vi "SaveResultToMES.vi"(0 "class data in":refnum<class "CMESAPI.lvclass">, 5 "serialNumber":string, 7 "equipment":string, 11 "error in (no error)":errorcluster) -> (4 "class data out":refnum<class "CMESAPI.lvclass">, 6 "Result":bool, 15 "error out":errorcluster)   [LabVIEW 2020, in "Salcomp-MES.lvlib" / "CMESAPI.lvclass"]
uses:
  CMESAPI.lvclass
  <vilib>/gpm_packages/@cs/event-logger/Source/Composed Log/Types/Log Level.ctl
  CMESAPI.lvclass/CMESAPI.ctl
  E:/Git/Libraries/develop/CME-API/CMESAPI_Fw4.0_1.9.2/CMESAPI.dll
  CMESAPI_Fw4.0_1.9.2/CMESAPI.dll
  <vilib>/gpm_packages/@cs/event-logger/Source/Composed Log/LoggerReference/LoggerReference.lvclass/LoggerReference.ctl
  <vilib>/gpm_packages/@cs/event-logger/Source/Composed Log/LoggerReference/Log.vi
  <vilib>/gpm_packages/@cs/event-logger/Source/Composed Log/LoggerReference/Get Valid Event Time.vi
  <vilib>/gpm_packages/@cs/event-logger/Source/Composed Log/LoggerReference/Remove Stale Logs.vi
  <vilib>/gpm_packages/@cs/event-logger/Source/Composed Log/LoggerReference/LoggerReference.lvclass
  <vilib>/gpm_packages/@cs/event-logger/Source/Composed Log/Composed Log.lvlib
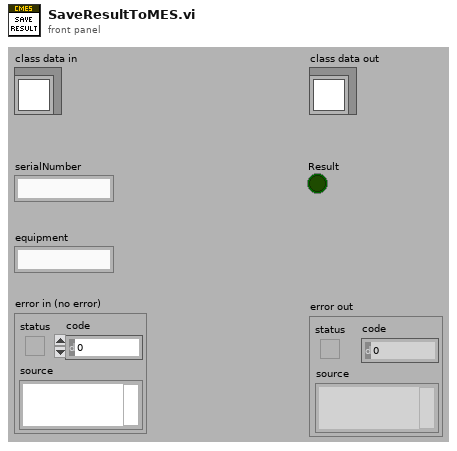
[diagram p1: front panel]
types:
  T1 = typedef "Composed Log.lvlib/Log Level.ctl" = enum16{"Debug", "Info", "Warning", "Error", "Critical"}
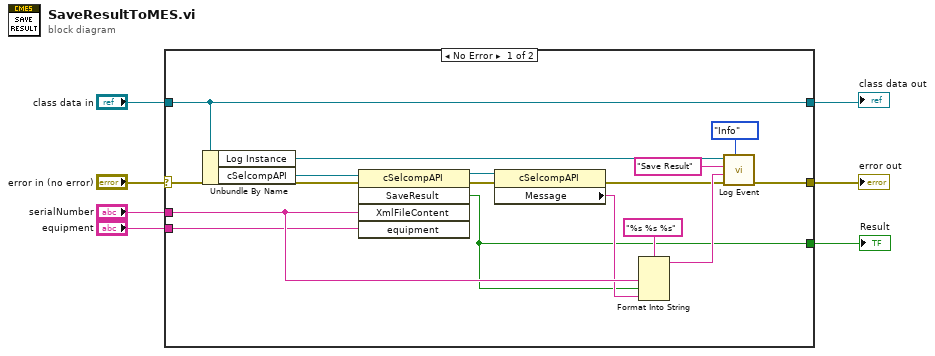
[diagram p0: block diagram]
diagram:
  n1 = case shown="No Error" "error in (no error)" {
    selector: "error in (no error)" -> [w21 w25]
    tunnel: [w15 w25] -> w6
    tunnel: "class data in" -> [w23 w24]
    tunnel: [w23 w24] -> w4
    tunnel: "serialNumber" -> [w11 _]
    tunnel: [w9 _] -> w1
    tunnel: "equipment" -> [w8 _]
    frame No Error {
      n2 = Unbundle By Name(w23) -> ("Log Instance"=w14:refnum<class "LoggerReference.lvclass">, "cSelcompAPI"=w22:refnum<k24>)
      n3 = invoke on="Invoke Node" class="cSelcompAPI" method="SaveResult"(reference=w22, error in=w21, "XmlFileContent"=w11, "equipment"=w8) -> (reference out=w12:refnum<k24>, error out=w16:errorcluster, "SaveResult"=w9:bool)  [unwired: 1 in, 2 out]
      n4 = property class="cSelcompAPI"(reference=w12, error in=w16) -> (error out=w13:errorcluster, "Message"=w10:string)  [unwired: 1 out]
      n5 = Format Into String(format string="%s %s %s", w11, w9, w10) -> (resulting string=w18:string)  [unwired: 2 in, 1 out]
      n6 = call <vilib>:"Log Event.vi"("Event Level"=Log_Level."Info", "error in (no error)"=w13, "Data To Log"=w18, "SourceID"="Save Result", "Log Instance"=w14) -> ("error out"=w15:errorcluster)  [unwired: 5 in, 1 out]
    }
    frame Error {
    }
  }
  "error out" <- w6
  "class data out" <- w4
  "Result" <- w1
